vi "Analysis.Result Summaries, First and Last Pass Yield Paretos_V2a.vi"(11 "ResultSum":T1[](array[typedef])) -> (2 "Test Count Table":string[][](table), 3 "Failure Pareto":string[][](table))   [LabVIEW 2024]
uses:
  Analysis.Result Summary_V2.ctl
  Analysis.Fail Paredo Gen Input_V2.ctl
panel:
  out "Tst Cnts":i32
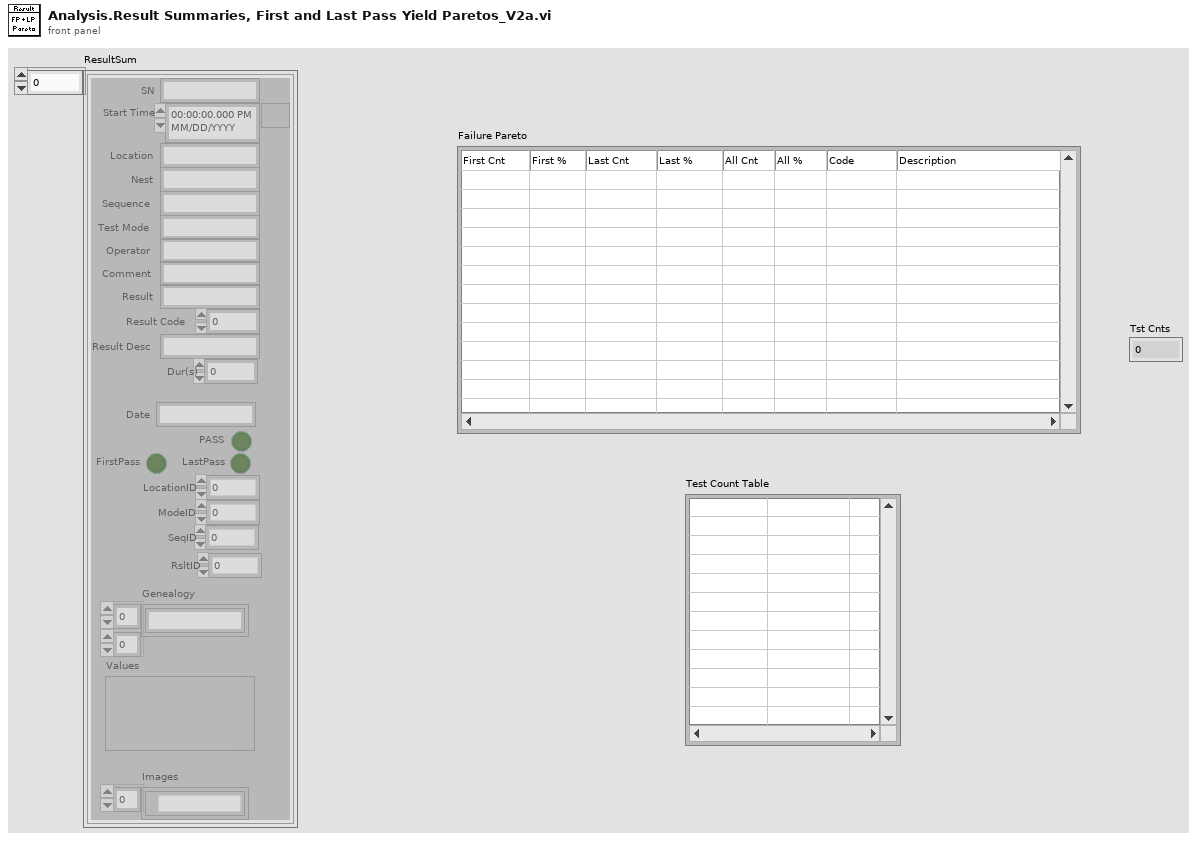
[diagram p1: front panel]
types:
  T1 = typedef "Analysis.Result Summary_V2.ctl" = cluster{"SN":string, "Start Time":timestamp, "Location":string, "Nest":string, "Sequence":string, "Operator":string, "Test Mode":string, "Comment":string, "Result":string, "Result Code":i32, "Result Desc":string, "Date":string, "Dur(s)":dbl, "PASS":bool, "FirstPass":bool, "LastPass":bool, "LocationID":i32, "ModeID":i32, "SeqID":i32, "RsltID":i32, "Genealogy":string[][], "Values":variant, "Images":path[]}
  T2 = typedef "Analysis.Fail Paredo Gen Input_V2.ctl" = cluster{"FirstPass":bool, "LastPass":bool, "Code":i32, "Desc":string, "Time":timestamp, "Loc":string}
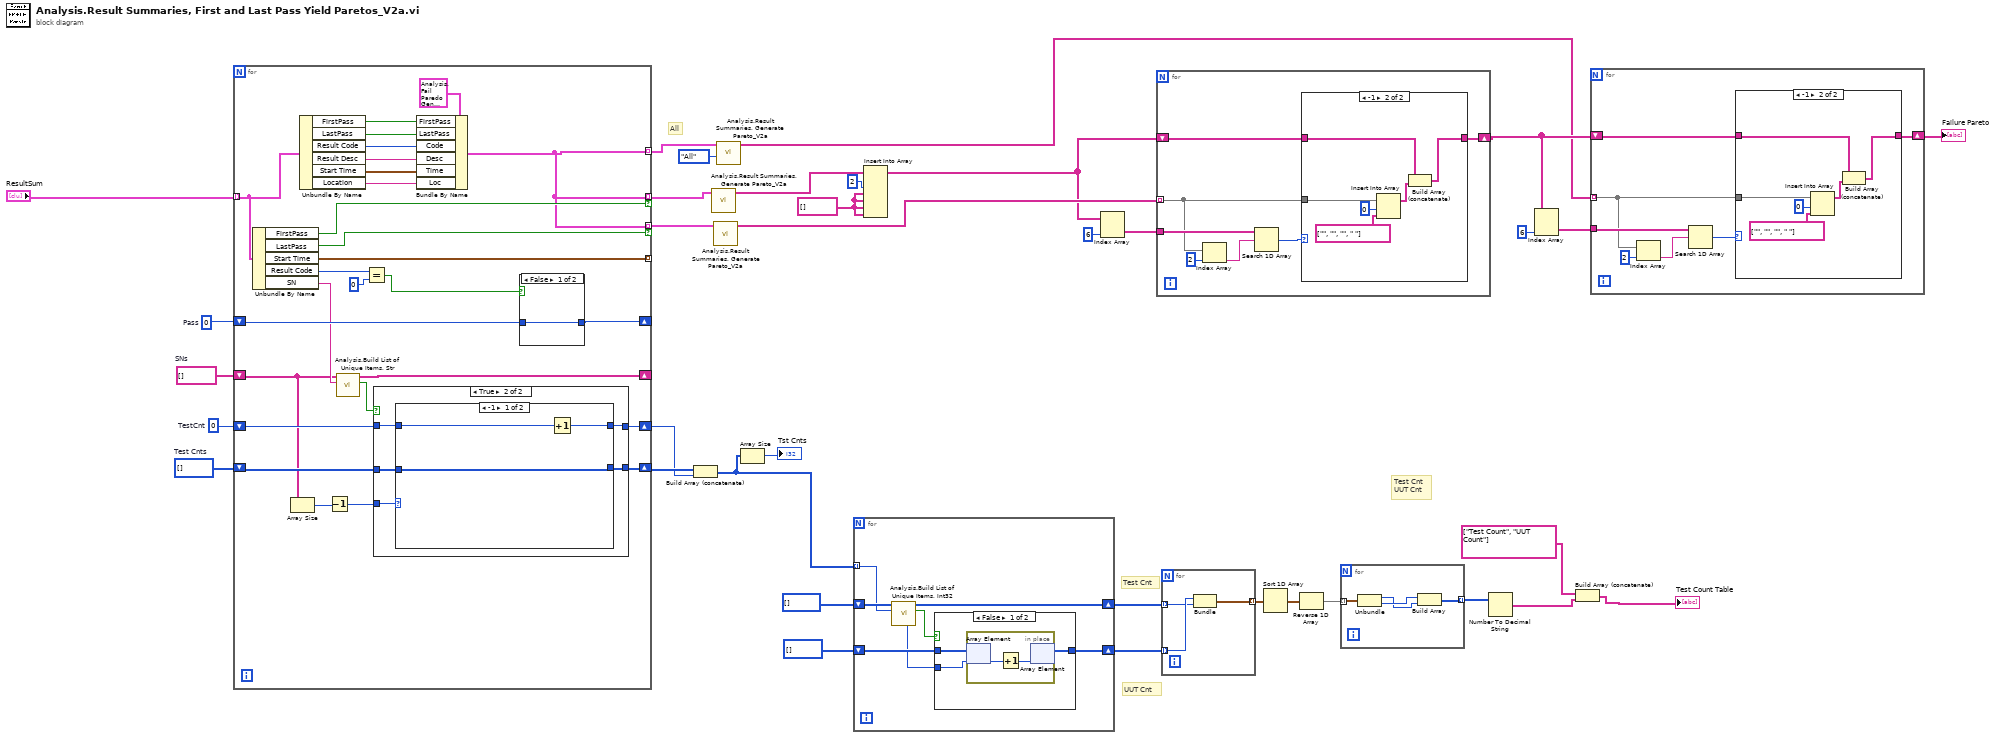
[diagram p0: block diagram]
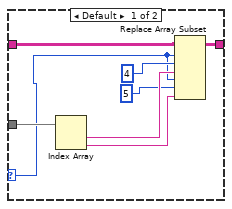
[diagram p2: hidden frame]
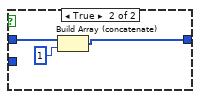
[diagram p3: hidden frame]
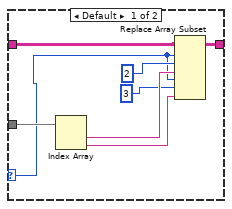
[diagram p4: hidden frame]
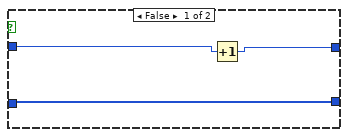
[diagram p5: hidden frame]
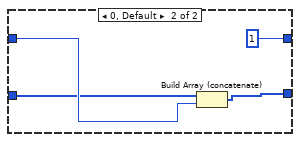
[diagram p6: hidden frame]
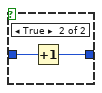
[diagram p7: hidden frame]
diagram:
  w10 = string[] []
  w32 = string[] []  # SNs
  w34 = i32[] []  # Test Cnts
  w33 = 0  # TestCnt
  w35 = 0  # Pass
  # "All"
  # "Test Cnt\nUUT Cnt"
  # "Test Cnt"
  # "UUT Cnt"
  n1 = for {
    tunnel: "ResultSum" -> [w44] mode=indexing
    tunnel: [w37] -> w4 mode=indexing if=w63
    tunnel: [w37] -> w36 mode=indexing if=w62
    tunnel: [w61] -> _ mode=indexing
    shift-right: [w58] -> _
    shift-left: w35 -> [w56]
    shift-right: [w50] -> w31
    shift-left: w34 -> [w52]
    shift-right: [w51] -> w30
    shift-left: w33 -> [w49]
    shift-right: [w54] -> _
    shift-left: w32 -> [w48]
    tunnel: [w37] -> w2 mode=indexing
    n2 = Unbundle By Name(w44) -> ("FirstPass"=w63:bool, "LastPass"=w62:bool, "Start Time"=w61:timestamp, "Result Code"=w60:i32, "SN"=w55:string)
    n3 = Array Size(array=w48) -> (size(s)=w47:i32)
    n4 = Unbundle By Name(w44) -> ("FirstPass"=w38:bool, "LastPass"=w39:bool, "Result Code"=w40:i32, "Result Desc"=w41:string, "Start Time"=w42:timestamp, "Location"=w43:string)
    n5 = Decrement(x=w47) -> (x-1=w46:i32)
    n6 = call "Analysis.Build List of Unique Items, Str.vi"("Item In"=w55, "List In"=w48) -> ("Added"=w53:bool, "List Out"=w54:string[])  [unwired: 7 in, 1 out]
    n7 = Equal?(x=w60, y=0) -> (x = y?=w57:bool)
    n8 = case shown="True" w53 {
      tunnel: w52 -> [w66 w68]
      tunnel: w49 -> [w65 w69]
      tunnel: [w64 w71] -> w51
      tunnel: [w66 w70] -> w50
      tunnel: w46 -> [_ w67]
      frame False {
        n9 = Increment(x=w65) -> (x+1=w64:i32)
      }
      frame True {
        n10 = case shown="-1" w67 {
          tunnel: [w72 1] -> w71
          tunnel: [w74 w77] -> w70
          tunnel: w69 -> [w73 w76]
          tunnel: w68 -> [w74 w75]
          frame -1 {
            n11 = Increment(x=w73) -> (x+1=w72:i32)
          }
          frame 0, Default {
            n12 = Build Array (concatenate)(w75, w76) -> (w77:i32[])
          }
        }
      }
    }
    n13 = Bundle By Name(cluster=T2 {"FirstPass"=FALSE, "LastPass"=FALSE, "Code"=0, "Desc"="", "Time"=timestamp(0 s since 1904-01-01), "Loc"=""} ("Pareto Gen Input"), "FirstPass"=w38, "LastPass"=w39, "Code"=w40, "Desc"=w41, "Time"=w42, "Loc"=w43) -> (w37:T2)
    n14 = case shown="False" w57 {
      tunnel: w56 -> [w79 w81]
      tunnel: [w79 w80] -> w58
      frame False {
      }
      frame True {
        n15 = Increment(x=w81) -> (x+1=w80:i32)
      }
    }
  }
  n16 = Build Array (concatenate)(w31, w30) -> (w22:i32[])
  n17 = call "Analysis.Result Summaries, Generate Pareto_V2a.vi"("ResultSum"=w4) -> ("FP Pareto"=w27:string[][])  [unwired: 10 in]
  n18 = call "Analysis.Result Summaries, Generate Pareto_V2a.vi"("ResultSum"=w36) -> ("FP Pareto"=w28:string[][])  [unwired: 10 in]
  n19 = call "Analysis.Result Summaries, Generate Pareto_V2a.vi"("Type"=enum16{"All", "FP", "LP"}."All", "ResultSum"=w2) -> ("FP Pareto"=w5:string[][])  [unwired: 9 in]
  n20 = Array Size(array=w22) -> (size(s)=→"Tst Cnts":i32)
  n21 = for {
    tunnel: w22 -> [w86] mode=indexing
    shift-right: [w87] -> w19
    shift-left: i32[] [] ("Test Cnts") -> [w88]
    shift-right: [w83] -> w18
    shift-left: i32[] [] ("Test Cnts") -> [w84]
    n22 = call "Analysis.Build List of Unique Items, Int32.vi"("Item In"=w86, "List In"=w88) -> ("Added"=w85:bool, "List Out"=w87:i32[], "Index"=w82:i32)  [unwired: 7 in]
    n23 = case shown="False" w85 {
      tunnel: w84 -> [w91 w95]
      tunnel: [w90 w96] -> w83
      tunnel: w82 -> [w89 _]
      frame False {
        n24 = in-place {
          n25 = in-place-array #1(w91, w89) -> (w93:i32)
          n26 = Increment(x=w93) -> (x+1=w92:i32)
          n27 = in-place-array #1(w92) -> (w90:i32[])  [unwired: 1 out]
        }
      }
      frame True {
        n28 = Build Array (concatenate)(w95, 1) -> (w96:i32[])
      }
    }
  }
  n29 = Insert Into Array(array=w27, index (col)=2 ("index (row)"), new element #1=w10, new element #2=w10, new element #3=w10, new element #4=w10) -> (w26:string[][])  [unwired: 1 in]
  n30 = Index Array(array=w26, index (col)=6 ("index (row)")) -> (element=w24:string[])  [unwired: 1 in]
  n31 = for {
    tunnel: w28 -> [w98] mode=indexing
    tunnel: w24 -> [w102]
    shift-right: [w97] -> w6
    shift-left: w26 -> [w100]
    n32 = Index Array(array=w98, index=2) -> (element=w101:string)
    n33 = Search 1D Array(1D array=w102, element=w101) -> (index of element=w99:i32)  [unwired: 1 in]
    n34 = case shown="-1" w99 {
      selector: w99 -> [w106 _]
      tunnel: w100 -> [w109 w117]
      tunnel: w98 -> [w111 w116]
      tunnel: [w110 w112] -> w97
      frame Default {
        n35 = Index Array(array=w111) -> (element #1=w107:string, element #2=w104:string)  [unwired: 2 in]
        n36 = Replace Array Subset(array=w109, new element #1=w107, index (row) #1=w106, index (col) #1=2 ("disabled index (col)"), new element #2=w104, index (row) #2=w106, index (col) #2=3 ("disabled index (col)")) -> (w110:string[][])
      }
      frame -1 {
        n37 = Insert Into Array(array=w116, index=0, new element=string[] ["", "", "", " "]) -> (w113:string[])
        n38 = Build Array (concatenate)(w117, w113) -> (w112:string[][])
      }
    }
  }
  n39 = for {
    tunnel: w19 -> [w119] mode=indexing
    tunnel: w18 -> [w120] mode=indexing
    tunnel: [w118] -> w17 mode=indexing
    n40 = Bundle("TestCnt"=w120, "TestCnt"=w119) -> (w118:cluster{"TestCnt":i32, "TestCnt":i32})  [unwired: 1 in]
  }
  n41 = Sort 1D Array(array=w17) -> (sorted array=w16:cluster{"TestCnt":i32, "TestCnt":i32}[])
  n42 = Reverse 1D Array(array=w16) -> (reversed array=w15:cluster{"TestCnt":i32, "TestCnt":i32}[])
  n43 = for {
    tunnel: w15 -> [w124] mode=indexing
    tunnel: [w121] -> w14 mode=indexing
    n44 = Unbundle(w124) -> ("TestCnt"=w122:i32, "TestCnt"=w123:i32)
    n45 = Build Array(w123, w122) -> (w121:i32[])
  }
  n46 = Number To Decimal String(number=w14) -> (decimal integer string=w11:string[][])  [unwired: 1 in]
  n47 = Index Array(array=w6, index (col)=6 ("index (row)")) -> (element=w9:string[])  [unwired: 1 in]
  n48 = Build Array (concatenate)(string[] ["Test Count", "UUT Count"], w11) -> (→"Test Count Table":string[][])
  n49 = for {
    tunnel: w5 -> [w126] mode=indexing
    tunnel: w9 -> [w130]
    shift-right: [w125] -> w7
    shift-left: w6 -> [w128]
    n50 = Index Array(array=w126, index=2) -> (element=w129:string)
    n51 = Search 1D Array(1D array=w130, element=w129) -> (index of element=w127:i32)  [unwired: 1 in]
    n52 = case shown="-1" w127 {
      selector: w127 -> [w134 _]
      tunnel: w128 -> [w137 w145]
      tunnel: w126 -> [w139 w144]
      tunnel: [w138 w140] -> w125
      frame Default {
        n53 = Index Array(array=w139) -> (element #1=w135:string, element #2=w132:string)  [unwired: 2 in]
        n54 = Replace Array Subset(array=w137, new element #1=w135, index (row) #1=w134, index (col) #1=4 ("disabled index (col)"), new element #2=w132, index (row) #2=w134, index (col) #2=5 ("disabled index (col)")) -> (w138:string[][])
      }
      frame -1 {
        n55 = Insert Into Array(array=w144, index=0, new element=string[] ["", "", "", " "]) -> (w141:string[])
        n56 = Build Array (concatenate)(w145, w141) -> (w140:string[][])
      }
    }
  }
  "Failure Pareto" <- w7
